vi "ToolToTeeth - Copy.vi"(9 "ProgramName":string="5", 10 "FileText":string="\n", 11 "ToolId":string="5") -> (3 "output string":string)   [LabVIEW 2017]
panel:
  out "substring before match":string
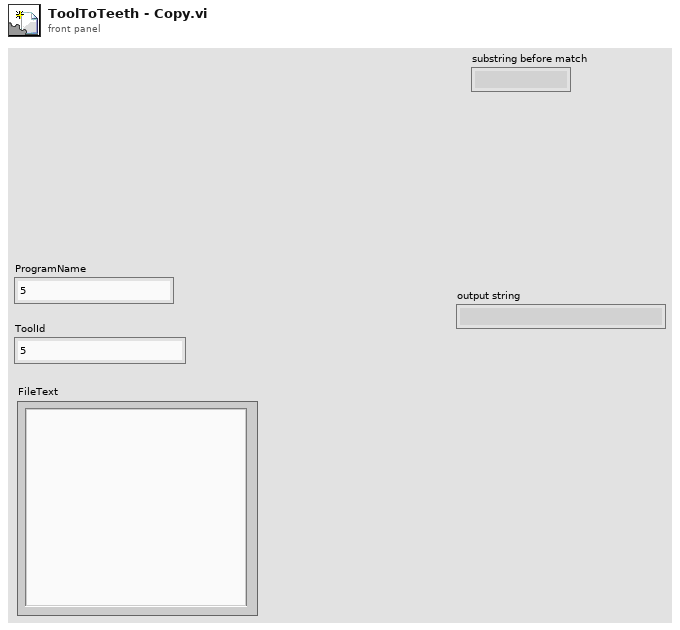
[diagram p1: front panel]
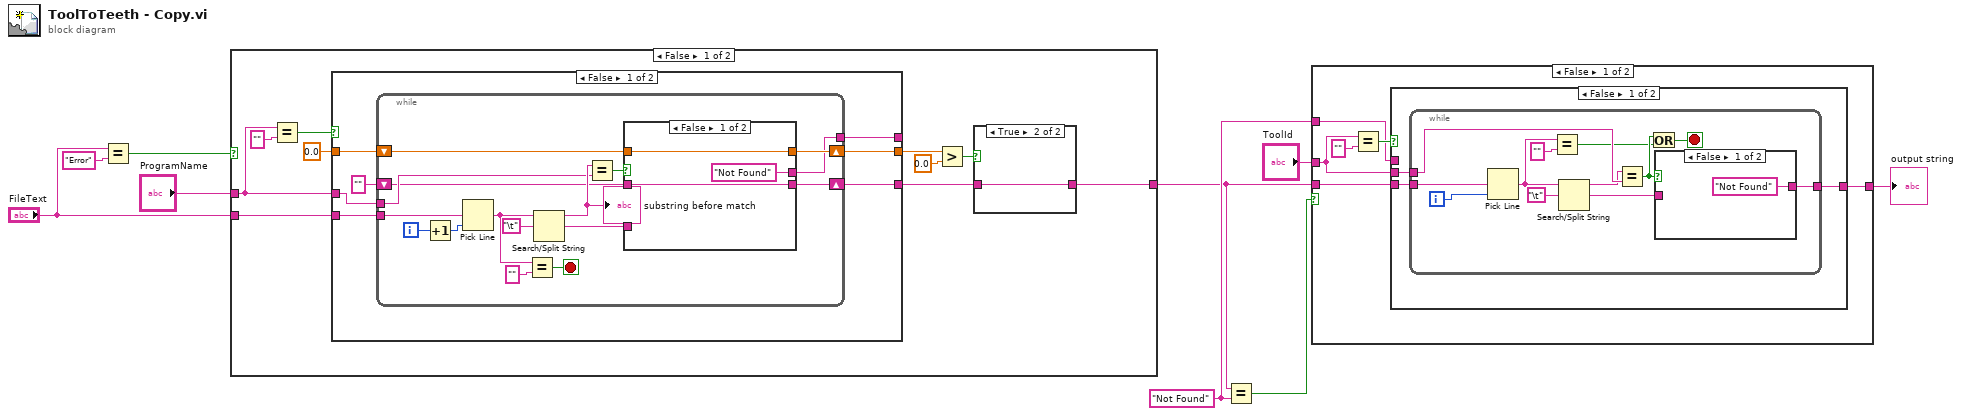
[diagram p0: block diagram]
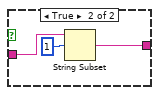
[diagram p2: hidden frame]
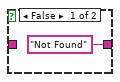
[diagram p5: hidden frame]
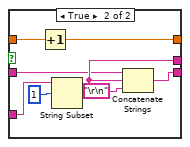
[diagram p6: hidden frame]
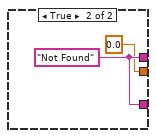
[diagram p7: hidden frame]
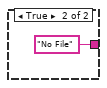
[diagram p8: hidden frame]
diagram:
  w5 = "Not Found"
  n1 = Equal?(x="FileText", y="Error") -> (x = y?=w7:bool)
  n2 = case shown="False" w7 {
    tunnel: "FileText" -> [w19 _]
    tunnel: "ProgramName" -> [w17 _]
    tunnel: [w10 "No File" ("output string")] -> w4
    frame False {
      n3 = Equal?(x=w17, y="") -> (x = y?=w16:bool)
      n4 = case shown="False" w16 {
        tunnel: w19 -> [w28 _]
        tunnel: [w27 w57] -> _
        tunnel: w17 -> [w26 _]
        tunnel: 0.0 -> [w25 _]
        tunnel: [w24 w57] -> w11
        tunnel: [w23 0.0] -> w14
        frame False {
          n5 = while {
            tunnel: w28 -> [w43]
            tunnel: w26 -> [w37]
            tunnel: [w32] -> w27
            shift-right: [w33] -> w23
            shift-left: w25 -> [w34]
            shift-right: [w31] -> w24
            shift-left: "" -> [w30]
            i -> [w39]
            stop <- w29 stop-if-true
            n6 = Increment(x=w39) -> (x+1=w40:i32)
            n7 = Pick Line(multi-line string=w43, line index=w40) -> (output string=w41:string)  [unwired: 1 in]
            n8 = Equal?(x=w41, y="") -> (x = y?=w29:bool)
            n9 = Search/Split String(string=w41, search string/char (-)="\t") -> (substring before match=w38:string, match + rest of string=w36:string)  [unwired: 1 in, 1 out]
            "substring before match" <- w38
            n10 = Equal?(x=w38, y=w37) -> (x = y?=w35:bool)
            n11 = case shown="False" w35 {
              tunnel: w36 -> [_ w54]
              tunnel: ["Not Found" ("output string") w51] -> w32
              tunnel: w34 -> [w46 w53]
              tunnel: [w46 w52] -> w33
              tunnel: [w45 w49] -> w31
              tunnel: w30 -> [w45 w48]
              frame False {
              }
              frame True {
                n12 = Increment(x=w53) -> (x+1=w52:dbl)
                n13 = String Subset(string=w54, offset (0)=1) -> (substring=w51:string)  [unwired: 1 in]
                n14 = Concatenate Strings(w48, w51, "\r\n") -> (w49:string)
              }
            }
          }
        }
        frame True {
          w57 = "Not Found" ("output string")
        }
      }
      n15 = Greater?(x=w14, y=0.0) -> (0:w12:bool)
      n16 = case shown="True" w12 {
        tunnel: w11 -> [_ w21]
        tunnel: ["Not Found" ("output string") w21] -> w10
        frame False {
        }
        frame True {
        }
      }
    }
    frame True {
    }
  }
  n17 = Equal?(x=w4, y=w5) -> (x = y?=w6:bool)
  n18 = case shown="False" w6 {
    tunnel: [w60 w85] -> w1
    tunnel: w5 -> [w59 w85]
    tunnel: w4 -> [w62 _]
    tunnel: "ToolId" -> [w61 _]
    frame False {
      n19 = Equal?(x=w61, y="") -> (x = y?=w63:bool)
      n20 = case shown="False" w63 {
        tunnel: w62 -> [w65 _]
        tunnel: [w67 w84] -> w60
        tunnel: w61 -> [w66 _]
        tunnel: w59 -> [_ w84]
        frame False {
          n21 = while {
            tunnel: w66 -> [w78]
            tunnel: w65 -> [w71]
            tunnel: [w79] -> w67
            i -> [w68]
            stop <- w69 stop-if-true
            n22 = Pick Line(multi-line string=w71, line index=w68) -> (output string=w70:string)  [unwired: 1 in]
            n23 = Equal?(x=w70, y="") -> (x = y?=w72:bool)
            n24 = Search/Split String(string=w70, search string/char (-)="\t") -> (substring before match=w75:string, match + rest of string=w74:string)  [unwired: 1 in, 1 out]
            n25 = Equal?(x=w75, y=w78) -> (x = y?=w73:bool)
            n26 = Or(x=w73, y=w72) -> (x .or. y?=w69:bool)
            n27 = case shown="False" w73 {
              tunnel: w74 -> [_ w82]
              tunnel: ["Not Found" ("output string") w81] -> w79
              frame False {
              }
              frame True {
                n28 = String Subset(string=w82, offset (0)=1) -> (substring=w81:string)  [unwired: 1 in]
              }
            }
          }
        }
        frame True {
        }
      }
    }
    frame True {
    }
  }
  "output string" <- w1
